vi "server.Wait for Request.vi"(8 "error in (no error)":errorcluster, 9 "timeout in ms (100)":i32=100, 11 "Server in":refnum<class "JSONRPC Server.lvclass">) -> (0 "error out":errorcluster, 1 "timed out?":bool, 2 "Request":refnum<class "Request.lvclass">, 3 "Server out":refnum<class "JSONRPC Server.lvclass">)   [LabVIEW 2016, in "JSONRPC Server.lvclass"]
doc: "This fetches a new request from the client.s"
uses:
  JSONRPC Server.lvclass
  Request/Request.lvclass
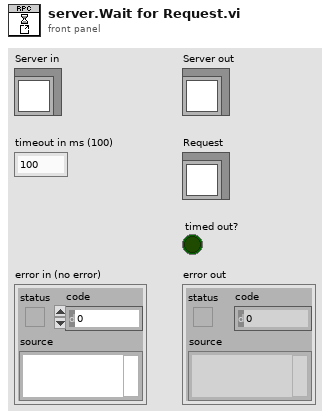
[diagram p1: front panel]
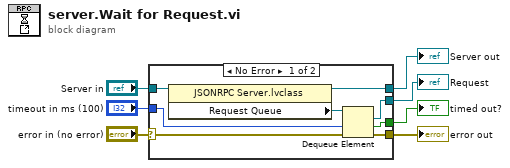
[diagram p0: block diagram]
diagram:
  n1 = case shown="No Error" "error in (no error)" {
    selector: "error in (no error)" -> [w14 w17]
    tunnel: [w12 w17] -> w6
    tunnel: [w9 w16] -> w4
    tunnel: "Server in" -> [w10 w16]
    tunnel: "timeout in ms (100)" -> [w15 _]
    tunnel: [w13 _] -> w2
    tunnel: [w11 _] -> w1
    frame No Error {
      n2 = property class="JSONRPC Server.lvclass"(reference=w10) -> (reference out=w9:refnum<class "JSONRPC Server.lvclass">, "Request Queue"=w8:refnum<queue>)  [unwired: 1 in, 1 out]
      n3 = Dequeue Element(queue=w8, timeout in ms (-1)=w15, error in (no error)=w14) -> (element=w13:refnum<class "Request.lvclass">, timed out?=w11:bool, error out=w12:errorcluster)  [unwired: 1 out]
    }
    frame Error {
    }
  }
  "error out" <- w6
  "Server out" <- w4
  "Request" <- w2
  "timed out?" <- w1
